vi "ConvertEZ-ZONEInputWords.vi"(11 "Word Array":u32[](array[numeric])) -> (3 "EZ-ZONE Input Cluster":T1={"Device Status"=0, "Analog Input Value 1"=0.0, "Analog Input Value 2"=0.0, "Heat Power"=0.0, "Cool Power"=0.0, "Profile Start"=0, "Current Profile"=0, "Current Step"=0, "Active Set Point"=0.0, "Step Time Remaining"=0, "Analog Input Error 1"=61, "Analog Input Error 2"=61, "Alarm State 1"=61, "Alarm State 2"=61, "Alarm State 3"=61, "Alarm State 4"=61, "Digital Input Status 5"=41, "Digital Input Status 6"=41, "Control Mode Active"=62, "Limit State"=62, "Profile Action Request"=61} {"Profile Action Request" items=["None"=61, "Start a Profile"=196, "Start a Step"=89, "Pause"=146, "Resume"=147, "End"=148]; "Limit State" items=["Off"=62, "None"=61, "Limit High"=51, "Limit Low"=52, "Error"=28]; "Control Mode Active" items=["Off"=62, "Auto"=10, "Manual"=54]; "Digital Input Status 6" items=["Inactive"=41, "Active"=5]; "Digital Input Status 5" items=["Inactive"=41, "Active"=5]; "Alarm State 4" items=["Startup"=88, "None"=61, "Blocked"=12, "Alarm Low"=8, "Alarm High"=7, "Error"=28]; "Alarm State 3" items=["Startup"=88, "None"=61, "Blocked"=12, "Alarm Low"=8, "Alarm High"=7, "Error"=28]; "Alarm State 2" items=["Startup"=88, "None"=61, "Blocked"=12, "Alarm Low"=8, "Alarm High"=7, "Error"=28]; "Alarm State 1" items=["Startup"=88, "None"=61, "Blocked"=12, "Alarm Low"=8, "Alarm High"=7, "Error"=28]; "Analog Input Error 2" items=["None"=61, "Open"=65, "Shorted"=127, "Measurement Error"=140, "Bad Calibration Data"=139, "Ambient Error"=9, "RTD Lead Resistance Error"=141]; "Analog Input Error 1" items=["None"=61, "Open"=65, "Shorted"=127, "Measurement Error"=140, "Bad Calibration Data"=139, "Ambient Error"=9, "RTD Lead Resistance Error"=141]})   [LabVIEW 2011]
uses:
  Controls/EZ-ZONE Input Cluster.ctl
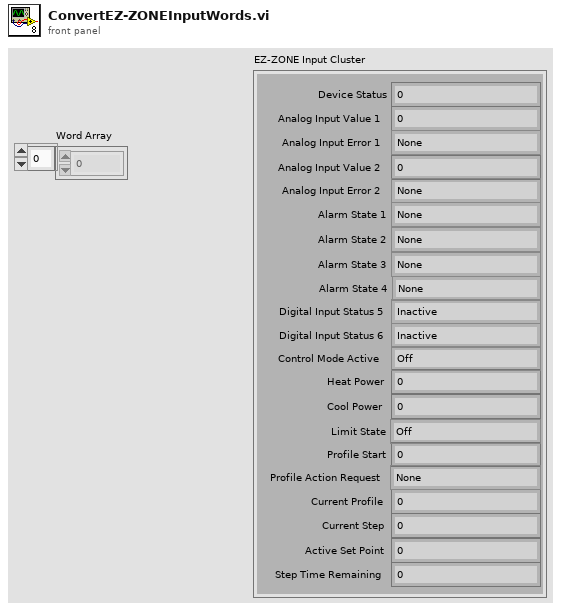
[diagram p1: front panel]
types:
  T1 = typedef "EZ-ZONE Input Cluster.ctl" = cluster{"Device Status":u32, "Analog Input Value 1":sgl, "Analog Input Value 2":sgl, "Heat Power":sgl, "Cool Power":sgl, "Profile Start":u32, "Current Profile":u32, "Current Step":u32, "Active Set Point":sgl, "Step Time Remaining":u32, "Analog Input Error 1":u32, "Analog Input Error 2":u32, "Alarm State 1":u32, "Alarm State 2":u32, "Alarm State 3":u32, "Alarm State 4":u32, "Digital Input Status 5":u32, "Digital Input Status 6":u32, "Control Mode Active":u32, "Limit State":u32, "Profile Action Request":u32}
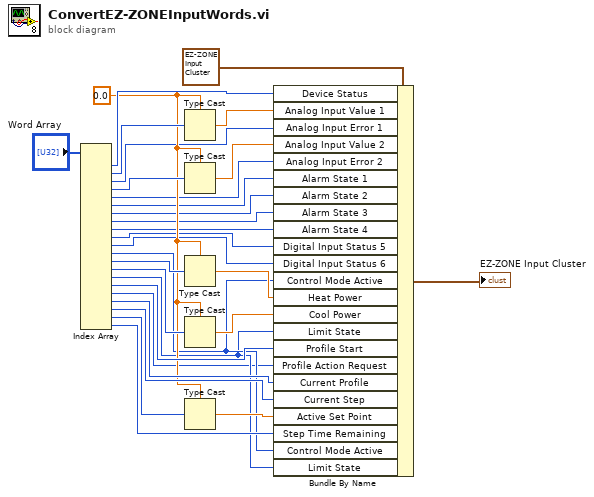
[diagram p0: block diagram]
diagram:
  w13 = sgl 0.0
  n1 = Index Array(array="Word Array") -> (element #1=w28:u32, element #2=w27:u32, element #3=w12:u32, element #4=w25:u32, element #5=w11:u32, element #6=w10:u32, element #7=w9:u32, element #8=w8:u32, element #9=w7:u32, element #10=w6:u32, element #11=w5:u32, element #12=w4:u32, element #13=w20:u32, element #14=w19:u32, element #15=w3:u32, element #16=w18:u32, element #17=w2:u32, element #18=w17:u32, element #19=w16:u32, element #20=w15:u32, element #21=w14:u32)  [unwired: 21 in]
  n2 = Type Cast(type=w13, x=w27) -> (*(type *) &x=w26:sgl)
  n3 = Type Cast(type=w13, x=w25) -> (*(type *) &x=w24:sgl)
  n4 = Type Cast(type=w13, x=w20) -> (*(type *) &x=w22:sgl)
  n5 = Type Cast(type=w13, x=w19) -> (*(type *) &x=w23:sgl)
  n6 = Type Cast(type=w13, x=w15) -> (*(type *) &x=w21:sgl)
  n7 = Bundle By Name(cluster=T1 {"Device Status"=0, "Analog Input Value 1"=0.0, "Analog Input Value 2"=0.0, "Heat Power"=0.0, "Cool Power"=0.0, "Profile Start"=0, "Current Profile"=0, "Current Step"=0, "Active Set Point"=0.0, "Step Time Remaining"=0, "Analog Input Error 1"=0, "Analog Input Error 2"=0, "Alarm State 1"=0, "Alarm State 2"=0, "Alarm State 3"=0, "Alarm State 4"=0, "Digital Input Status 5"=0, "Digital Input Status 6"=0, "Control Mode Active"=0, "Limit State"=0, "Profile Action Request"=0} ("EZ-ZONE Input Cluster"), "Device Status"=w28, "Analog Input Value 1"=w26, "Analog Input Error 1"=w12, "Analog Input Value 2"=w24, "Analog Input Error 2"=w11, "Alarm State 1"=w10, "Alarm State 2"=w9, "Alarm State 3"=w8, "Alarm State 4"=w7, "Digital Input Status 5"=w6, "Digital Input Status 6"=w5, "Control Mode Active"=w4, "Heat Power"=w22, "Cool Power"=w23, "Limit State"=w3, "Profile Start"=w18, "Profile Action Request"=w2, "Current Profile"=w17, "Current Step"=w16, "Active Set Point"=w21, "Step Time Remaining"=w14, "Control Mode Active"=w4, "Limit State"=w3) -> (→"EZ-ZONE Input Cluster":T1)
